vi "Manual Init.vi"(8 "error in":errorcluster, 10 "DeviceID":T1, 11 "SCADA in":refnum<class "EMS.lvclass">) -> (0 "error out":errorcluster, 3 "SCADA out":refnum<class "EMS.lvclass">)   [LabVIEW 2018, in "EMS Core.lvlib" / "EMS.lvclass"]
uses:
  EMS.lvclass
  C:/Users/Administrator/Desktop/LabVIEW EMS/EMS Generic Actor/EMS Generic/EMS Generic.lvclass
  C:/Program Files (x86)/National Instruments/LabVIEW 2018/vi.lib/ActorFramework/Actor/Actor.lvclass
  <vilib>/ORNL/CSEISMIC DDS/CSEISMIC DDS Base/Data Types/Controls/DeviceID.ctl
  Controls/Microgrid State.ctl
  EMS.lvclass/EMS.ctl
  <vilib>/ActorFramework/Message Enqueuer/Message Enqueuer.lvclass/Message Enqueuer.ctl
  <vilib>/ActorFramework/Actor/Actor.lvclass/Actor.ctl
  EMS Messages/Return Microgrid State Msg/Return Microgrid State Msg.lvclass/Return Microgrid State Msg.ctl
  <vilib>/ActorFramework/Message Enqueuer/Enqueue.vi
  <vilib>/ActorFramework/Stop Msg/Stop Msg.lvclass
  C:/Program Files (x86)/National Instruments/LabVIEW 2018/vi.lib/ActorFramework/Message/Message.lvclass
  EMS Messages/Return Microgrid State Msg/Return Microgrid State Msg.lvclass
  <vilib>/ActorFramework/Message Priority Queue/Priority Enqueue.vi
  <vilib>/ActorFramework/Actor/Actor.lvclass
  EMS Generic Actor/EMS Generic/EMS Generic.lvclass
  <vilib>/ORNL/CSEISMIC DDS/CSEISMIC DDS Base/CSEISMIC DDS.lvclass
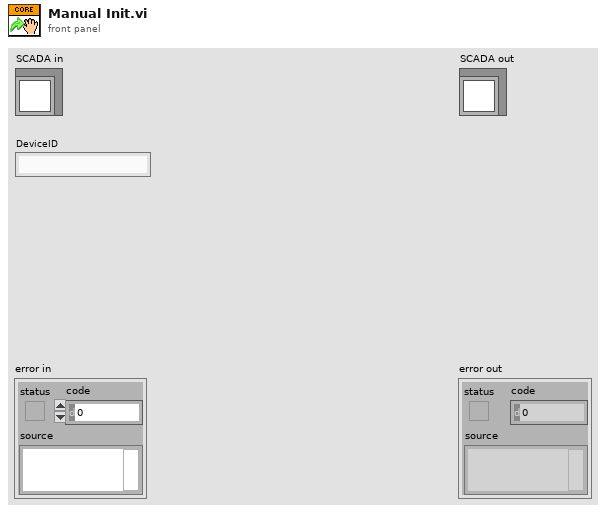
[diagram p1: front panel]
types:
  T1 = typedef "CSEISMIC DDS.lvlib/CSEISMIC DDS.lvclass/DeviceID.ctl" = string
  T2 = typedef "EMS Core.lvlib/EMS.lvclass/Microgrid State.ctl" = enum16{"Discovery", "Commissioning", "Activation", "Blackstart", "OnGrid", "OffGrid", "Island", "Resynchronization", "Manual", "Shutdown", "Stop"}
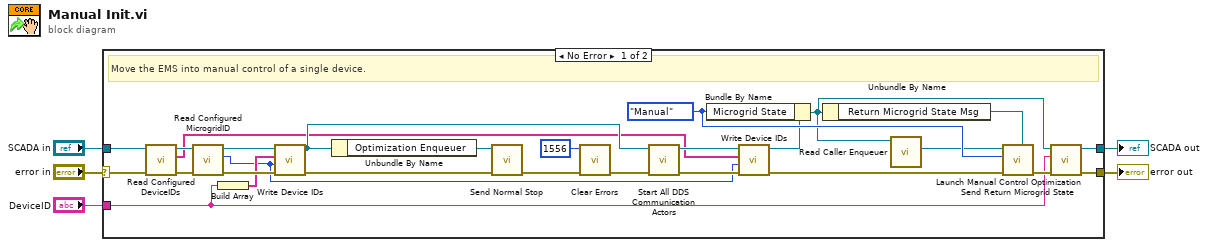
[diagram p0: block diagram]
diagram:
  n1 = case shown="No Error" "error in" {
    selector: "error in" -> [w16 w34]
    tunnel: [w24 w34] -> w4
    tunnel: [w25 w33] -> w2
    tunnel: "SCADA in" -> [w17 w33]
    tunnel: "DeviceID" -> [w19 _]
    frame No Error {
      w29 = Microgrid_State."Manual" ("Microgrid State")
      # "Move the EMS into manual control of a single device."
      n2 = call "Read Configured DeviceIDs.vi"("error in"=w16, "EMS Generic in"=w17) -> ("error out"=w15:errorcluster, "DeviceIDs"=w7:T1[], "EMS Generic out"=w12:refnum<class "EMS.lvclass">)  [unwired: 7 in]
      n3 = call "Read Configured MicrogridID.vi"("error in"=w15, "EMS Generic in"=w12) -> ("error out"=w21:errorcluster, "Microgrid ID"=w6:u8, "EMS Generic out"=w20:refnum<class "EMS.lvclass">)  [unwired: 7 in]
      n4 = Build Array(w19) -> (w18:T1[])
      n5 = call "Write Device IDs.vi"("error in"=w21, "Microgrid ID"=w6, "Device ID Array"=w18, "EMS Generic in"=w20) -> ("error out"=w22:errorcluster, "dup EMS Generic out"=w14:refnum<class "EMS.lvclass">)  [unwired: 6 in]
      n6 = Unbundle By Name(w14) -> ("Optimization Enqueuer"=w30:refnum<class "Message Enqueuer.lvclass">)
      n7 = call <vilib>:"Send Normal Stop.vi"("error in (no error)"=w22, "Message Enqueuer"=w30) -> ("error out"=w31:errorcluster)  [unwired: 9 in]
      n8 = call <vilib>:"Clear Errors.vi"("error in (no error)"=w31, "specific error code to clear (0: all)"=1556) -> ("error out"=w13:errorcluster)  [unwired: 4 in, 1 out]
      n9 = call "Start All DDS Communication Actors.vi"("error in"=w13, "SCADA in"=w14) -> ("error out"=w9:errorcluster, "SCADA out"=w11:refnum<class "EMS.lvclass">)  [unwired: 8 in]
      n10 = call "Write Device IDs.vi"("error in"=w9, "Microgrid ID"=w6, "Device ID Array"=w7, "EMS Generic in"=w11) -> ("error out"=w8:errorcluster, "dup EMS Generic out"=w10:refnum<class "EMS.lvclass">)  [unwired: 6 in]
      n11 = Bundle By Name(cluster=w10, "Microgrid State"=w29) -> (w26:refnum<class "EMS.lvclass">)
      n12 = Unbundle By Name(w26) -> ("Return Microgrid State Msg"=w28:refnum<class "Return Microgrid State Msg.lvclass">)
      n13 = call <vilib>:"Read Caller Enqueuer.vi"("Actor"=w26) -> ("Caller Enqueuer"=w27:refnum<class "Message Enqueuer.lvclass">)  [unwired: 10 in]
      n14 = call "Send Return Microgrid State.vi"("Message Type"=w28, "error in (no error)"=w8, "Microgrid State"=w29, "Message Enqueuer"=w27) -> ("error out"=w23:errorcluster)  [unwired: 6 in, 1 out]
      n15 = call "Launch Manual Control Optimization.vi"("error in"=w23, "DeviceID"=w19, "SCADA in"=w26) -> ("error out"=w24:errorcluster, "SCADA out"=w25:refnum<class "EMS.lvclass">)  [unwired: 7 in]
    }
    frame Error {
    }
  }
  "error out" <- w4
  "SCADA out" <- w2
